vi "Build.vi"(8 "error in (no error)":errorcluster, 11 "Build in":refnum<class "AB_Deploy_EXE.lvclass">) -> (0 "error out":errorcluster, 1 "GeneratedFiles":path[](array[path]), 2 "GeneratedDirectories":path[](array[path]), 3 "Build out":refnum<class "AB_Deploy_EXE.lvclass">, 4 "GeneratedFileGUIDs":string[](array[string]), 5 "OutputDirectory":path, 7 "Dependencies":T1[](array[typedef]))   [LabVIEW 2020, in "AB_Deploy_EXE.lvclass"]
uses:
  <vilib>/AppBuilder/AB_Classes/DeployableEXE/AB_Deploy_EXE.lvclass
  e:/builds/penguin/labview/branches/2020/dev/dist/vi.lib/AppBuilder/AB_Classes/Build/AB_Build.lvclass
  <vilib>/AppBuilder/AB_Dependency.ctl
  <vilib>/Utility/lvfile.llb/LVFileType.ctl
  <vilib>/AppBuilder/AB_Classes/DeployableEXE/AB_Deploy_EXE.lvclass/AB_Deploy_EXE.ctl
  <vilib>/AppBuilder/AB_Classes/EXE/AB_EXE.lvclass
  <vilib>/AppBuilder/AB_Classes/Destination/AB_Destination.lvclass
  <vilib>/AppBuilder/AB_Classes/Build/AB_Build.lvclass
  <vilib>/Utility/lvfile.llb/NI_FileType.lvlib
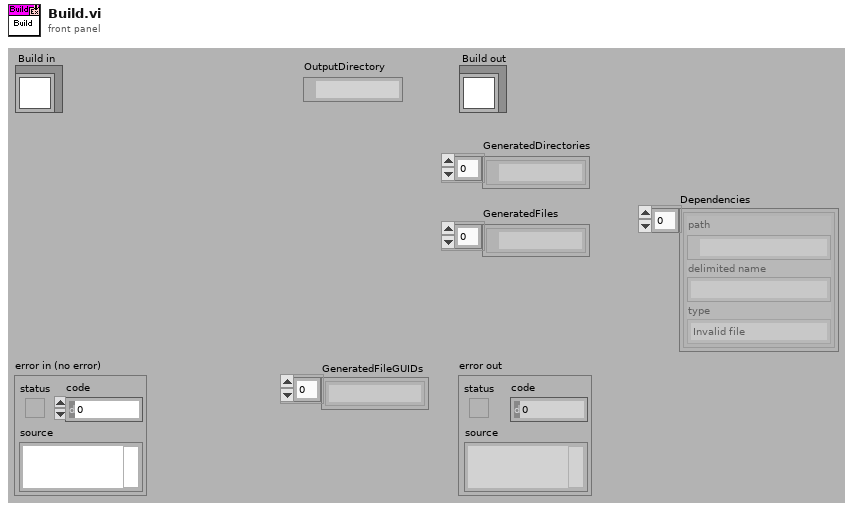
[diagram p1: front panel]
types:
  T1 = typedef "AB_Dependency.ctl" = cluster{"path":path, "delimited name":string, "type":T2}
  T2 = typedef "NI_FileType.lvlib/LVFileType.ctl" = enum32{"Invalid file", "Unknown type", "Instrument", "Control", "Polymorphic VI", "Project", "Library", "LVClass", "XControl", "XNode", "Shared library", ".NET assembly", "ActiveX interface", "CIN", "Run-time menu", "Palette menu", "Help file", "LLB", "XNode Edit Dependency", "Class Private Data Control", "Statechart", "MathScript .m file", "Ladder Diagram", "LVLibp", "XNode Build Dependency"}
  T3 = typedef "AB_Build.ctl" = cluster{"buildSpecName":string, "buildSpecDescription":string, "destinations":refnum<class "AB_Destination.lvclass">[], "exclusionOption":T4, "defaultLanguage":string, "supportedLanguages":string[], "excludedDirectories":path[], "buildContext":refnum<vi>, "buildObject":T5, "preview":bool, "programatic":bool, "progressBarEvents":T6, "userLog_Path":path, "preActionID":string, "preAction_Path":path, "postActionID":string, "postAction_Path":path, "eng_checkForBrokenVIs?":bool, "eng_verboseLinkerErrors?":bool, "localDest_Path":path, "targetDest_Path":path, "removeVIObject":u16, "cache":refnum<class "PreviewCache.lvclass">, "use cache":bool, "previewCache_ID":string, "buildCache_ID":string, "eng_TempLocalDest_Path":path, "eng_collectDependencies?":bool, "versionInfo":cluster{"buildVersion":cluster{"major":u16, "minor":u16, "patch":u16, "build":u16}, "autoIncrement":bool}, "eng_enableVIChecksums":bool}
  T4 = typedef "AB_Exclusion_Option.ctl" = cluster{"typedefs":bool, "polymorphicVIs":bool, "unusedLibraryItems":bool, "modifyLibraryFile":bool, "edit-timeDependencies":bool, "inlineVIs":bool, "dependent PPLs":bool, "dependent DLLs":bool}
  T5 = typedef "ItemRef.ctl" = u64
  T6 = typedef "provcom_ProgressBar_Events.ctl" = cluster{"newJob":refnum<user-event>, "newItem":refnum<user-event>, "errorMsg":T7, "cancel":refnum<user-event>}
  T7 = typedef "mxLvBuildError.ctl" = refnum<user-event>
  T8 = typedef "AB_Destination.ctl" = cluster{"destName":string, "path":path, "libraryName":string, "preserveHierarchy":bool, "eng_inBuild":bool, "eng_libraryReference":refnum<vi>, "eng_restictAddToNewLibrary":bool}
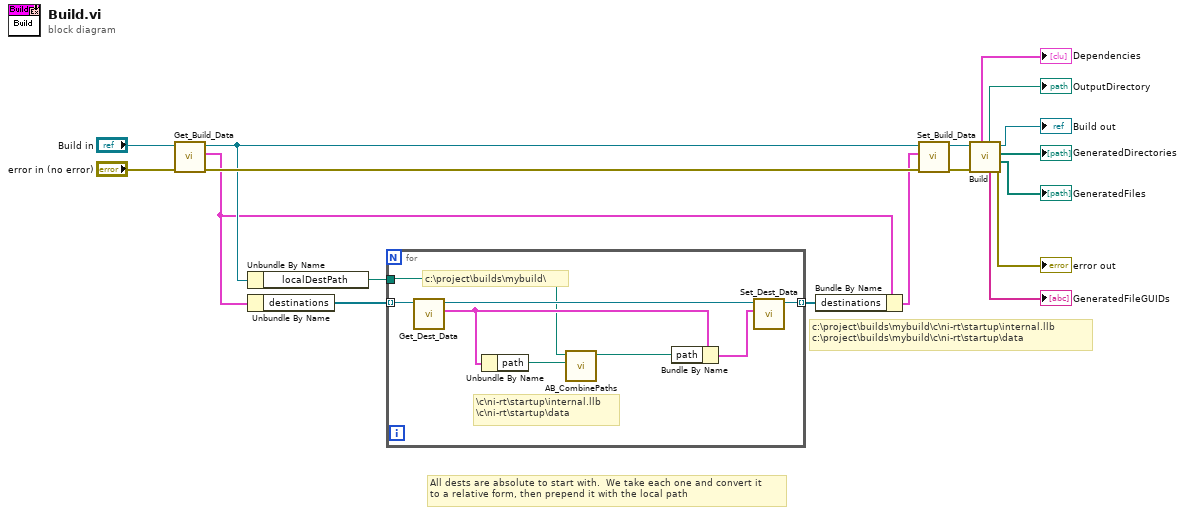
[diagram p0: block diagram]
diagram:
  # "c:\\project\\builds\\mybuild\\c\\ni-rt\\startup\\internal.llb\nc:\\project\\builds\\mybuild\\c\\ni-rt\\startup\\data"
  # "All dests are absolute to start with.  We take each one and convert it\nto a relative form, then prepend it with the local path"
  n1 = call <vilib>:"Get_Build_Data.vi"("error in (no error)"="error in (no error)", "Class in"="Build in") -> ("error out"=w12:errorcluster, "data"=w8:T3, "Class out"=w11:refnum<class "AB_Deploy_EXE.lvclass">)  [unwired: 7 in]
  n2 = Unbundle By Name(w11) -> ("localDestPath"=w6:path)
  n3 = Unbundle By Name(w8) -> ("destinations"=w7:refnum<class "AB_Destination.lvclass">[])
  n4 = for {
    tunnel: w7 -> [w26] mode=indexing
    tunnel: w6 -> [w20]
    tunnel: [w22] -> w10 mode=indexing
    # "\\c\\ni-rt\\startup\\internal.llb\n\\c\\ni-rt\\startup\\data"
    # "c:\\project\\builds\\mybuild\\"
    n5 = call <vilib>:"Get_Dest_Data.vi"("Class in"=w26) -> ("destName"=w25:T8, "Class out"=w24:refnum<class "AB_Destination.lvclass">)  [unwired: 8 in, 1 out]
    n6 = Unbundle By Name(w25) -> ("path"=w21:path)
    n7 = call <vilib>:"AB_CombinePaths.vi"("target path"=w21, "localDestPath"=w20) -> ("combined path"=w19:path)  [unwired: 9 in]
    n8 = Bundle By Name(cluster=w25, "path"=w19) -> (w23:T8)
    n9 = call <vilib>:"Set_Dest_Data.vi"("destName"=w23, "Class in"=w24) -> ("Class out"=w22:refnum<class "AB_Destination.lvclass">)  [unwired: 8 in, 1 out]
  }
  n10 = Bundle By Name(cluster=w8, "destinations"=w10) -> (w9:T3)
  n11 = call <vilib>:"Set_Build_Data.vi"("error in (no error)"=w12, "data"=w9, "Class in"=w11) -> ("error out"=w2:errorcluster, "Class out"=w4:refnum<class "AB_Deploy_EXE.lvclass">)  [unwired: 7 in]
  n12 = call-parent "Build.vi"("error in (no error)"=w2, "Build in"=w4) -> ("error out"=→"error out":errorcluster, "GeneratedFiles"=→"GeneratedFiles":path[], "GeneratedDirectories"=→"GeneratedDirectories":path[], "Build out"=→"Build out":refnum<class "AB_Deploy_EXE.lvclass">, "GeneratedFileGUIDs"=→"GeneratedFileGUIDs":string[], "OutputDirectory"=→"OutputDirectory":path, "Dependencies"=→"Dependencies":T1[])  [unwired: 3 in]
